vi "find most recent vip build.vi"(11 "VIPB file":path) -> (1 "search spec":string, 2 "found":bool, 3 "most recent build":path)   [LabVIEW 2010]
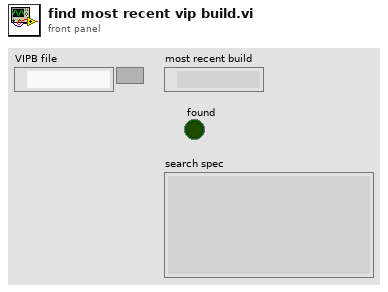
[diagram p1: front panel]
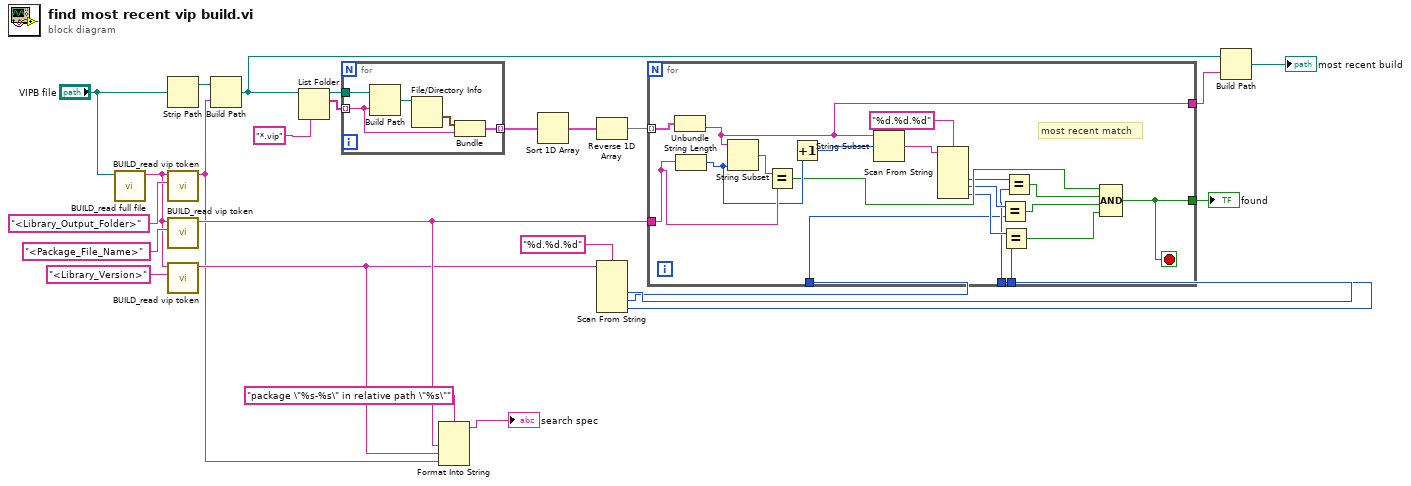
[diagram p0: block diagram]
diagram:
  n1 = call "BUILD_read full file.vi"("vip file"="VIPB file") -> ("data"=w8:string)  [unwired: 9 in, 1 out]
  n2 = Strip Path(path="VIPB file") -> (stripped path=w6:path)  [unwired: 1 out]
  n3 = call "BUILD_read vip token.vi"("regular expression"="<Library_Output_Folder>", "data"=w8) -> ("trimmed string"=w2:string)  [unwired: 9 in]
  n4 = call "BUILD_read vip token.vi"("regular expression"="<Package_File_Name>", "data"=w8) -> ("trimmed string"=w4:string)  [unwired: 9 in]
  n5 = call "BUILD_read vip token.vi"("regular expression"="<Library_Version>", "data"=w8) -> ("trimmed string"=w3:string)  [unwired: 9 in]
  n6 = Build Path(base path=w6, name or relative path=w2) -> (appended path=w14:path)
  n7 = List Folder(path=w14, pattern="*.vip") -> (path out=w24:path, filenames=w23:string[])  [unwired: 2 in, 2 out]
  n8 = for {
    tunnel: w24 -> [w30]
    tunnel: w23 -> [w27] mode=indexing
    tunnel: [w26] -> w22 mode=indexing
    n9 = Build Path(base path=w30, name or relative path=w27) -> (appended path=w29:path)
    n10 = File/Directory Info(path=w29) -> (last mod=w28:timestamp)  [unwired: 1 in, 6 out]
    n11 = Bundle("last mod"=w28, w27) -> (w26:cluster{"last mod":timestamp, string})  [unwired: 1 in]
  }
  n12 = Format Into String(format string="package \"%s-%s\" in relative path \"%s\"", w4, w3, w2) -> (resulting string=→"search spec":string)  [unwired: 2 in, 1 out]
  n13 = Sort 1D Array(array=w22) -> (sorted array=w21:cluster{"last mod":timestamp, string}[])
  n14 = Reverse 1D Array(array=w21) -> (reversed array=w20:cluster{"last mod":timestamp, string}[])
  n15 = Scan From String(format string="%d.%d.%d", input string=w3) -> (output 1=w18:i32, output 2=w17:i32, output 3=w16:i32)  [unwired: 5 in, 3 out]
  n16 = for {
    tunnel: w20 -> [w49] mode=indexing
    tunnel: w4 -> [w47]
    tunnel: w18 -> [w35]
    tunnel: w17 -> [w34]
    tunnel: w16 -> [w33]
    tunnel: [w32] -> w15
    tunnel: [w31] -> w13
    stop <- w31 stop-if-true
    # "most recent match"
    n17 = Unbundle(w49) -> (w32:string)  [unwired: 1 out]
    n18 = String Length(string=w47) -> (length=w45:i32)
    n19 = String Subset(string=w32, length (rest)=w45) -> (substring=w48:string)  [unwired: 1 in]
    n20 = Equal?(x=w48, y=w47) -> (x = y?=w42:bool)
    n21 = Increment(x=w45) -> (x+1=w46:i32)
    n22 = String Subset(string=w32, offset (0)=w46) -> (substring=w44:string)  [unwired: 1 in]
    n23 = Scan From String(format string="%d.%d.%d", input string=w44) -> (output 1=w38:i32, output 2=w37:i32, output 3=w36:i32)  [unwired: 5 in, 3 out]
    n24 = Equal?(x=w37, y=w34) -> (x = y?=w40:bool)
    n25 = Equal?(x=w36, y=w33) -> (x = y?=w39:bool)
    n26 = Equal?(x=w38, y=w35) -> (x = y?=w41:bool)
    n27 = Compound Arithmetic op=AND(w42, w41, w40, w39) -> (w31:bool)
  }
  "found" <- w13
  n28 = Build Path(base path=w14, name or relative path=w15) -> (appended path=→"most recent build":path)
